vi "EVM_ProgressBar.vi"(6 "Max 100? (T)":bool=TRUE, 8 "Goal points":u32, 9 "Current points":u32) -> (0 "Progress Caption Text":string="0%", 1 "Progress Value":dbl)   [LabVIEW 2010, in "lib1299.lvlib"]
doc: "This VI formats the status of the progress meter.\n\nInputs:\nCurrent points - current number of points collected\nGoal points - desired number of points to collected\n\nOutputs:\nProgress value - progress bar value\nProgress Caption Text - progress bar caption text"
uses:
  lib1299.lvlib
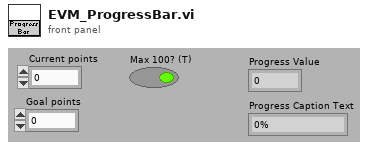
[diagram p1: front panel]
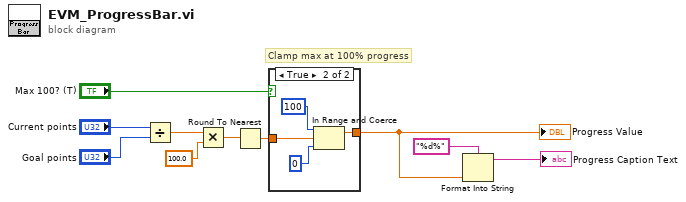
[diagram p0: block diagram]
diagram:
  # "Clamp max at 100% progress"
  n1 = Divide(x="Current points", y="Goal points") -> (x/y=w9:dbl)
  n2 = Multiply(x=w9, y=100.0) -> (x*y=w10:dbl)
  n3 = Round To Nearest(number=w10) -> (nearest integer value=w5:dbl)
  n4 = case shown="True" "Max 100? (T)" {
    tunnel: w5 -> [w11 w15]
    tunnel: [w11 w12] -> w3
    frame False {
    }
    frame True {
      n5 = In Range and Coerce(upper limit=100, x=w15, lower limit=0) -> (coerced(x)=w12:dbl)  [unwired: 1 out]
    }
  }
  "Progress Value" <- w3
  n6 = Format Into String(format string="%d%" ("path"), w3) -> (resulting string=→"Progress Caption Text":string)  [unwired: 2 in, 1 out]
